vi "MultiselectListboxStimulus.vi"(11 "error in (no error)":errorcluster) -> (15 "error out":errorcluster)   [LabVIEW 2016, in "DronaTest.lvlib"]
uses:
  DronaTest.lvlib
  APIs/Stimulus/ControlValue/SetValueAuto.vi
  APIs/Stimulus/ControlValue/Controls/Listbox/SetValueByArrayIndex.vi
  APIs/Assert/AssertControlValue/Equal.vi
  APIs/Stimulus/ControlValue/Controls/Listbox/SetValueByArrayName.vi
  APIs/Stimulus/VI/CloseVI.vi
  <vilib>/addons/_JKI Toolkits/Caraya/classes/Test/Test.lvclass
  Drona.lvlib
  <vilib>/SLL Toolkit/SLL Debug/SLL Debug.lvlib
  APIs/Assert/AssertControlValue/AssertControlValue.lvlib
  APIs/Stimulus/ControlValue/ControlValue.lvlib
  APIs/Stimulus/VI/VI.lvlib
  APIs/Stimulus/ControlValue/Controls/Listbox/Listbox.lvlib
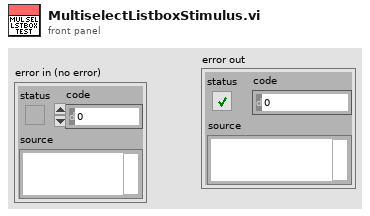
[diagram p1: front panel]
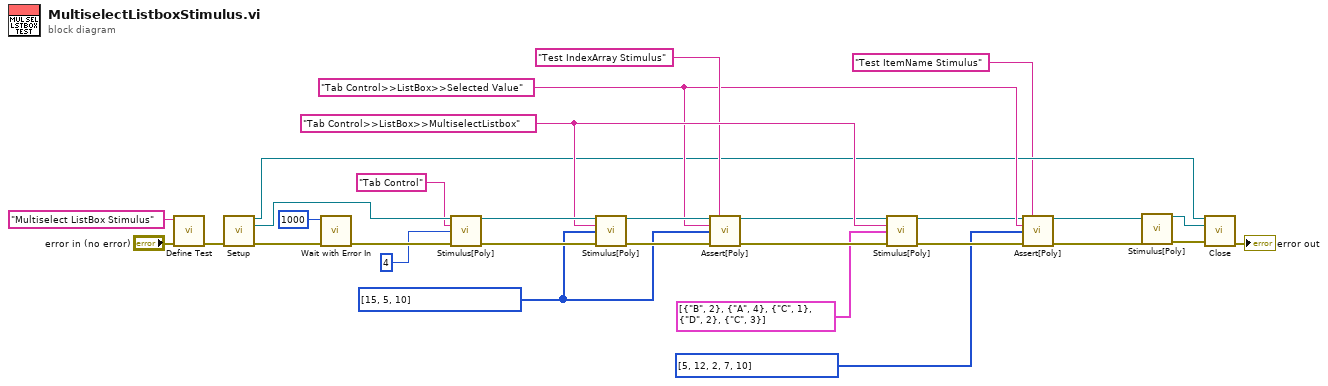
[diagram p0: block diagram]
diagram:
  w5 = i32[] [15, 5, 10] ("Index Array")
  w12 = "Tab Control>>ListBox>>Selected Value" ("Control Path")
  w18 = "Tab Control>>ListBox>>MultiselectListbox" ("Control Path")
  n1 = call <vilib>:"Define Test.vi"("error in (no error)"="error in (no error)", "Label (VI Title)"="Multiselect ListBox Stimulus") -> ("error out"=w29:errorcluster)  [unwired: 9 in]
  n2 = call "Setup.vi"("error in"=w29) -> ("Application Ref"=w7:refnum<vi>, "VI Reference Out"=w23:refnum<vi>, "error out"=w28:errorcluster)  [unwired: 12 in]
  n3 = call <vilib>:"Wait with Error In.vi"("error in (no error)"=w28, "milliseconds to wait"=u32 1000) -> ("error out"=w25:errorcluster)  [unwired: 9 in]
  n4 = call-poly "Stimulus[Poly].vi"("VI Reference In"=w23, "Control Path"="Tab Control", "Value (Signaling)"=4, "error in"=w25) -> ("VI Reference Out"=w19:refnum<vi>, "error out"=w24:errorcluster)  [unwired: 10 in]
  n5 = call-poly "Stimulus[Poly].vi"("VI Reference In"=w19, "Control Path"=w18, "Index Array"=w5, "Error In"=w24) -> ("VI Reference Out"=w16:refnum<vi>, "Error Out"=w17:errorcluster)  [unwired: 10 in]
  n6 = call-poly "Assert[Poly].vi"("VI Reference In"=w16, "Test Label"="Test IndexArray Stimulus", "Control Path"=w12, "Control Value"=w5, "Error In"=w17) -> ("VI Reference Out"=w13:refnum<vi>, "Error Out"=w14:errorcluster)  [unwired: 9 in]
  n7 = call-poly "Stimulus[Poly].vi"("VI Reference In"=w13, "Control Path"=w18, "Name Array"=cluster{"ItemName":string, "Occurance":i32}[] [{"ItemName"="B", "Occurance"=2}, {"ItemName"="A", "Occurance"=4}, {"ItemName"="C", "Occurance"=1}, {"ItemName"="D", "Occurance"=2}, {"ItemName"="C", "Occurance"=3}], "Error In"=w14) -> ("VI Reference Out"=w3:refnum<vi>, "Error Out"=w4:errorcluster)  [unwired: 10 in]
  n8 = call-poly "Assert[Poly].vi"("VI Reference In"=w3, "Test Label"="Test ItemName Stimulus", "Control Path"=w12, "Control Value"=i32[] [5, 12, 2, 7, 10] ("Index Array"), "Error In"=w4) -> ("VI Reference Out"=w8:refnum<vi>, "Error Out"=w9:errorcluster)  [unwired: 9 in]
  n9 = call-poly "Stimulus[Poly].vi"("VI Reference In"=w8, "error in"=w9) -> ("VI Reference Out"=w11:refnum<vi>, "error out"=w10:errorcluster)  [unwired: 12 in]
  n10 = call "Close.vi"("Application Ref"=w7, "VI Reference"=w11, "error in"=w10) -> ("error out"=→"error out":errorcluster)  [unwired: 12 in]
